vi "Write NumberOfRobots.vi"(8 "error in (no error)":errorcluster, 10 "NumberOfRobots":dbl=2.0, 11 "NormalGamePlay in":refnum<class "NormalGamePlay.lvclass">) -> (0 "error out":errorcluster, 3 "NormalGamePlay out":refnum<class "NormalGamePlay.lvclass">)   [LabVIEW 2020, in "NormalGamePlay.lvclass"]
uses:
  NormalGamePlay.lvclass
  NormalGamePlay.lvclass/NormalGamePlay.ctl
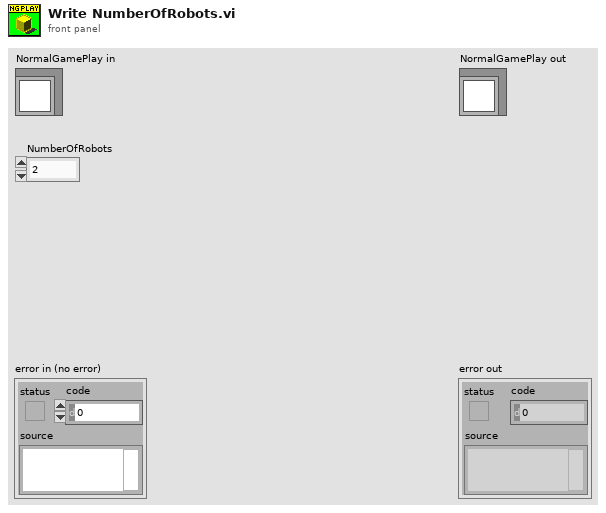
[diagram p1: front panel]
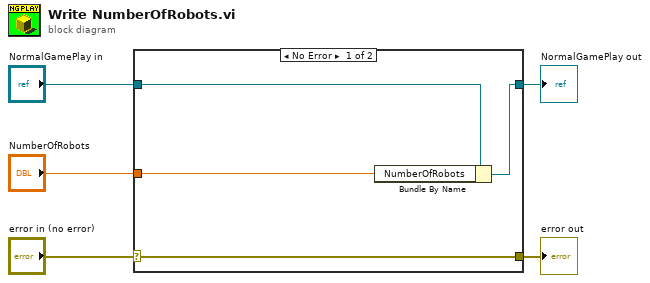
[diagram p0: block diagram]
diagram:
  n1 = case shown="No Error" "error in (no error)" {
    selector: "error in (no error)" -> [w9 w10]
    tunnel: [w9 w10] -> w4
    tunnel: [w7 w11] -> w2
    tunnel: "NormalGamePlay in" -> [w8 w11]
    tunnel: "NumberOfRobots" -> [w6 _]
    frame No Error {
      n2 = Bundle By Name(cluster=w8, "NumberOfRobots"=w6) -> (w7:refnum<class "NormalGamePlay.lvclass">)
    }
    frame Error {
    }
  }
  "error out" <- w4
  "NormalGamePlay out" <- w2
